vi "XYGraphTableTlog.vi"(0 "NouvTemps":dbl, 1 "XData":dbl[](array[numeric]) caption="Tous les temps", 5 "Max Index":i32, 7 "NouvDonnées Y":dbl[](array[numeric]), 9 "Actual Point Index":i32, 11 "error in (no error)":errorcluster, 12 "All YData":dbl[][](array[numeric]), 13 "TracerCourbe":bool[](array[boolean])) -> (3 "XData Out":dbl[](array[numeric]) caption="Tous les temps Out", 6 "XYGraph":T1(array[cluster]), 14 "All YData out":dbl[][](array[numeric]), 15 "error out":errorcluster)   [LabVIEW 2010]
doc: "Ce Vi ajoute les nouvelles données acquisitionner dans les tables de toutes les données acquisitionner. Il formate ensuite les données sous forme de cluster pour l'affichage dans un graphique XY."
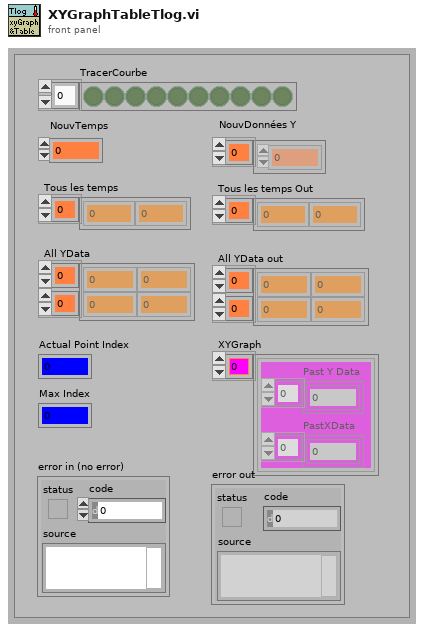
[diagram p1: front panel]
types:
  T1 = cluster{"Past Y Data":dbl[], "PastXData":dbl[]}[]
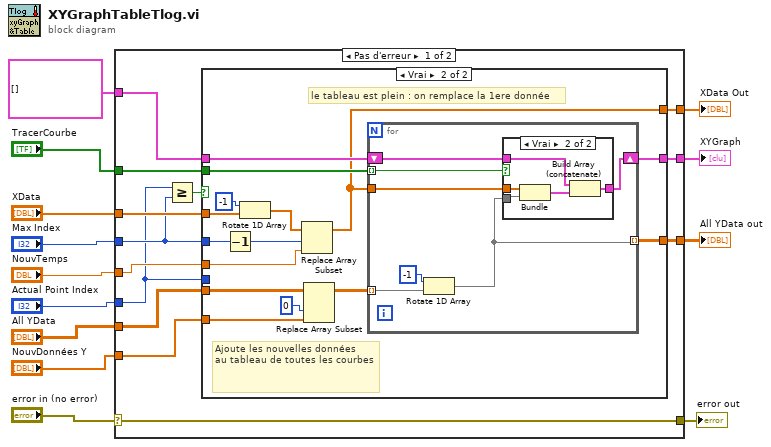
[diagram p0: block diagram]
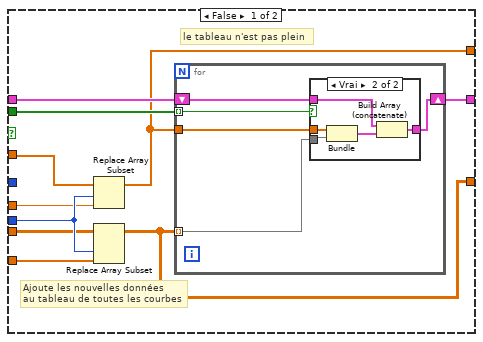
[diagram p2: hidden frame]
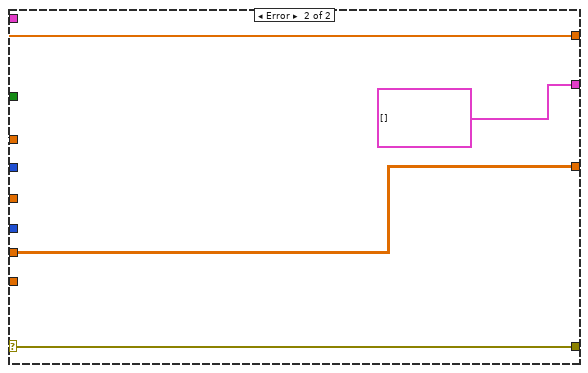
[diagram p5: hidden frame]
diagram:
  n1 = case shown="Pas d'erreur" "error in (no error)" {
    selector: "error in (no error)" -> [w23 w79]
    tunnel: "NouvDonnées Y" -> [w17 _]
    tunnel: "XData" -> [w20 w76]
    tunnel: "NouvTemps" -> [w19 _]
    tunnel: "Actual Point Index" -> [w15 _]
    tunnel: "All YData" -> [w18 w77]
    tunnel: [w26 cluster{"XData":dbl[], "All YData":dbl[]}[] []] -> w8
    tunnel: [w23 w79] -> w9
    tunnel: [w21 w77] -> w7
    tunnel: [w22 w76] -> w6
    tunnel: "TracerCourbe" -> [w25 _]
    tunnel: T1 [] ("XYGraph In") -> [w24 _]
    tunnel: "Max Index" -> [w16 _]
    frame No Error {
      n2 = Greater Or Equal?(x=w15, y=w16) -> (x >= y?=w14:bool)
      n3 = case shown="Vrai" w14 {
        tunnel: [w36 w62] -> w26
        tunnel: w25 -> [w35 w61]
        tunnel: w24 -> [w34 w60]
        tunnel: [w28 w48] -> w22
        tunnel: [w27 w59] -> w21
        tunnel: w20 -> [w33 w54]
        tunnel: w16 -> [_ w53]
        tunnel: w19 -> [w31 w52]
        tunnel: w18 -> [w30 w51]
        tunnel: w17 -> [w29 w50]
        tunnel: w15 -> [w32 _]
        frame False {
          # "le tableau n'est pas plein"
          # "Ajoute les nouvelles données\nau tableau de toutes les courbes"
          n4 = Replace Array Subset(array=w33, new element=w31, index=w32) -> (w28:dbl[])
          n5 = Replace Array Subset(array=w30, new element=w29, index (col)=w32) -> (w27:dbl[][])  [unwired: 1 in]
          n6 = for {
            tunnel: w28 -> [w41]
            tunnel: w35 -> [w39] mode=indexing
            shift-right: [w40] -> w36
            shift-left: w34 -> [w38]
            tunnel: w27 -> [w37] mode=indexing
            n7 = case shown="Vrai" w39 {
              tunnel: w41 -> [_ w47]
              tunnel: [w42 w46] -> w40
              tunnel: w38 -> [w42 w45]
              tunnel: w37 -> [_ w44]
              frame False {
              }
              frame True {
                n8 = Bundle("XData"=w47, "All YData"=w44) -> (w43:cluster{"XData":dbl[], "All YData":dbl[]})  [unwired: 1 in]
                n9 = Build Array (concatenate)(w45, w43) -> (w46:cluster{"XData":dbl[], "All YData":dbl[]}[])
              }
            }
          }
        }
        frame True {
          # "le tableau est plein : on remplace la 1ere donnée"
          # "Ajoute les nouvelles données\nau tableau de toutes les courbes"
          n10 = Decrement(x=w53) -> (x-1=w56:i32)
          n11 = Rotate 1D Array(1:w54, 2:-1 ("n")) -> (0:w57:dbl[])
          n12 = Replace Array Subset(array=w57, new element=w52, index=w56) -> (w48:dbl[])
          n13 = Replace Array Subset(array=w51, new element=w50, index (col)=0 ("disabled index (col)")) -> (w49:dbl[][])  [unwired: 1 in]
          n14 = for {
            tunnel: w48 -> [w69]
            tunnel: w61 -> [w67] mode=indexing
            shift-right: [w68] -> w62
            shift-left: w60 -> [w66]
            tunnel: w49 -> [w65] mode=indexing
            tunnel: [w64] -> w59 mode=indexing
            n15 = Rotate 1D Array(1:w65, 2:-1 ("n")) -> (0:w64:dbl[])
            n16 = case shown="Vrai" w67 {
              tunnel: w69 -> [_ w75]
              tunnel: [w70 w74] -> w68
              tunnel: w66 -> [w70 w73]
              tunnel: w64 -> [_ w72]
              frame False {
              }
              frame True {
                n17 = Bundle(w75, w72) -> (w71:cluster{dbl[], dbl[]})  [unwired: 1 in]
                n18 = Build Array (concatenate)(w73, w71) -> (w74:T1)
              }
            }
          }
        }
      }
    }
    frame Error {
    }
  }
  "error out" <- w9
  "XYGraph" <- w8
  "All YData out" <- w7
  "XData Out" <- w6
